vi "PositioningSet_FGV.vi"(0 "In":dbl[](array[numeric]), 2 "FGV_Control":enum16{"Set", "Get"}(ring), 5 "error in":errorcluster) -> (14 "out":dbl[](array[numeric]), 19 "error out":errorcluster)   [LabVIEW 2011]
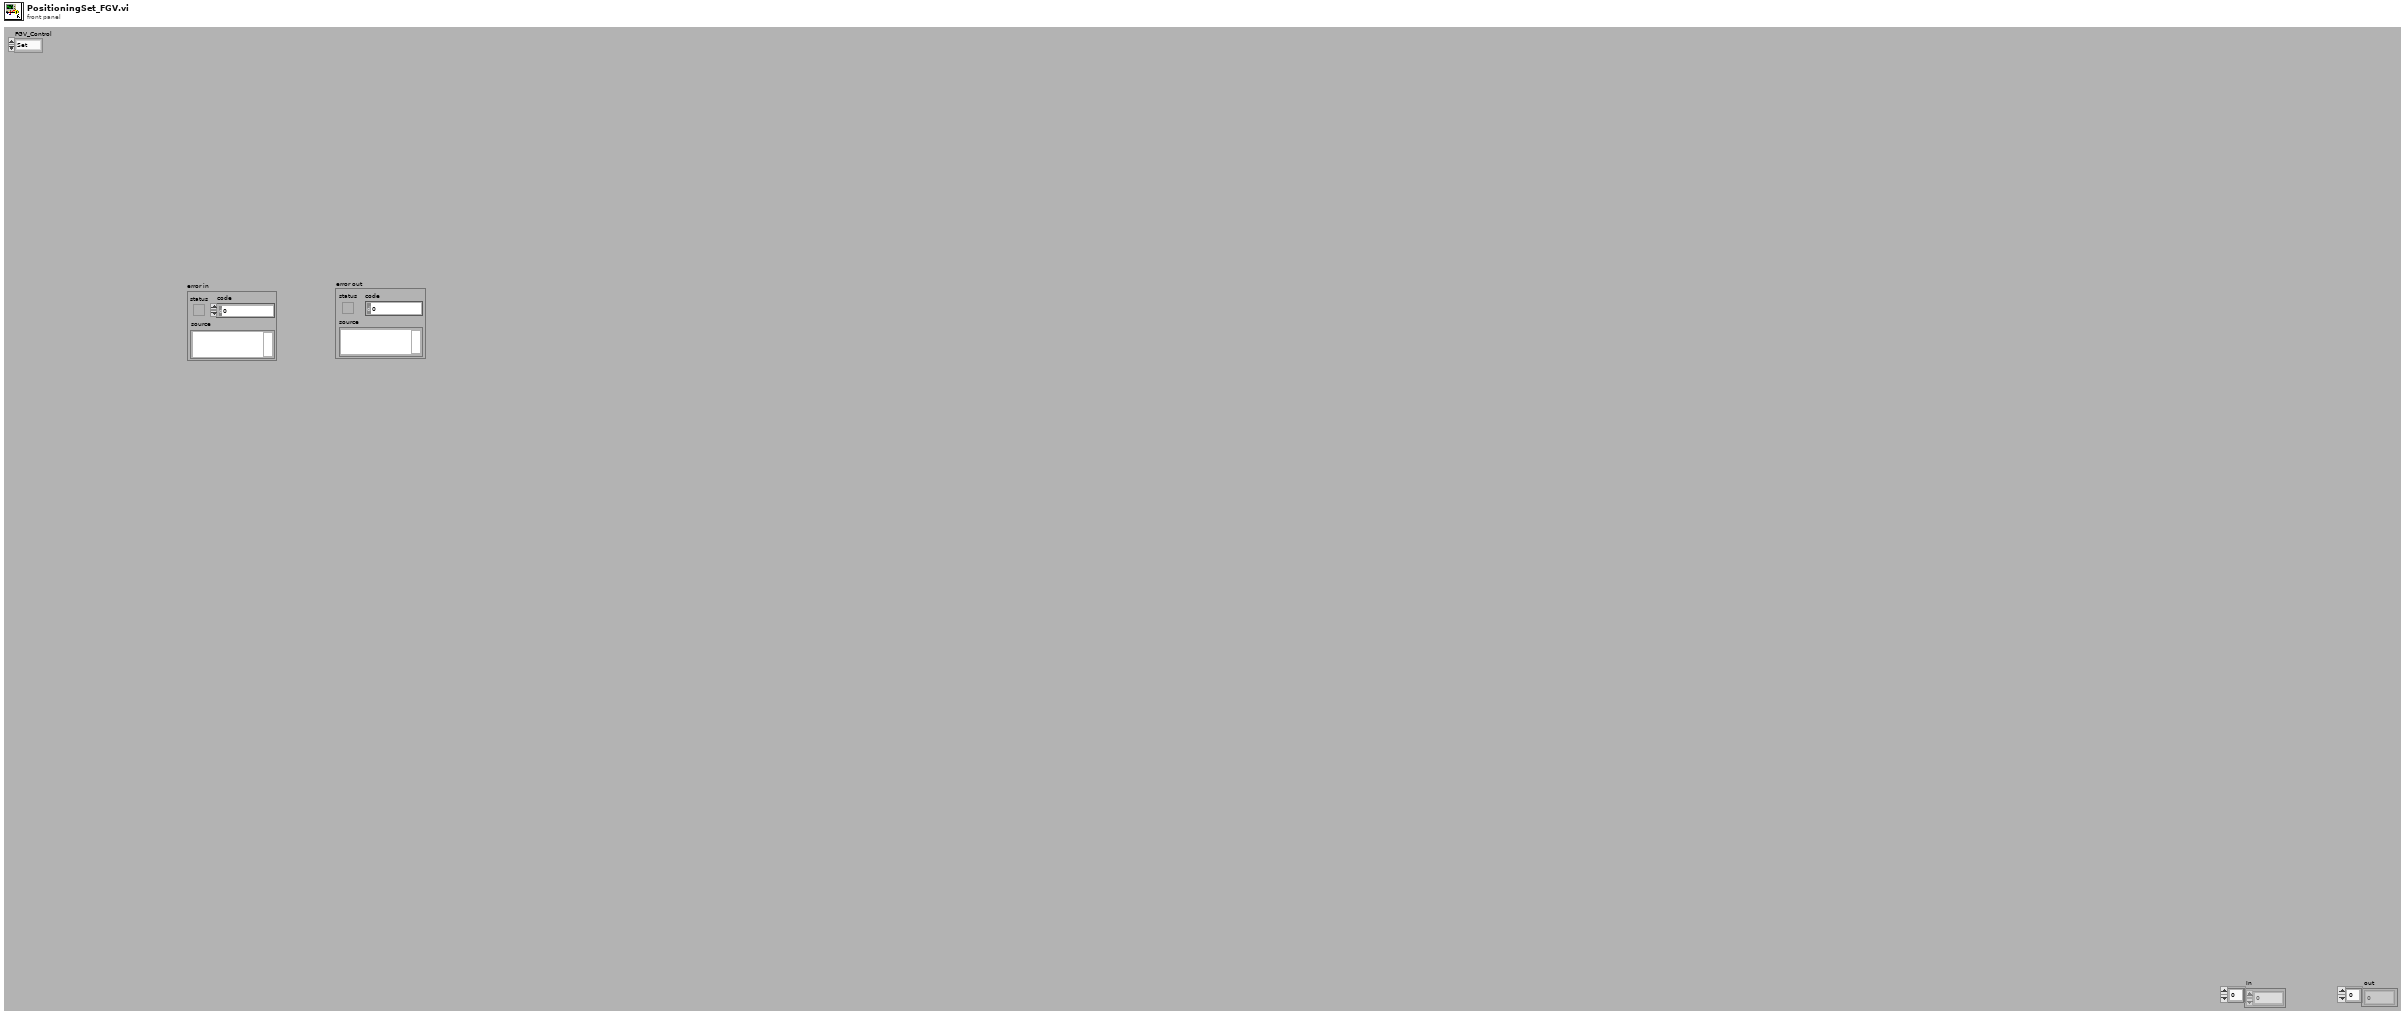
[diagram p1: front panel]
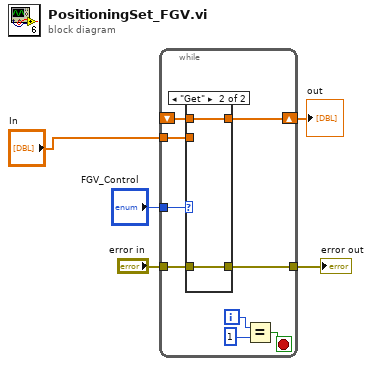
[diagram p0: block diagram]
diagram:
  n1 = while {
    tunnel: "In" -> [w14]
    shift-right: [w13] -> w1
    shift-left: _ -> [w12]
    tunnel: "error in" -> [w8]
    tunnel: [w7] -> w4
    tunnel: "FGV_Control" -> [w6]
    i -> [w9]
    stop <- w10 stop-if-true
    n2 = case shown="\"Get\"" w6 {
      tunnel: w14 -> [w16 _]
      tunnel: [w16 w18] -> w13
      tunnel: w12 -> [_ w18]
      tunnel: w8 -> [w15 w17]
      tunnel: [w15 w17] -> w7
      frame "Set", Default {
      }
      frame "Get" {
      }
    }
    n3 = Equal?(x=w9, y=1) -> (x = y?=w10:bool)
  }
  "error out" <- w4
  "out" <- w1
